vi "json_resolve_key.vi"(11 "key":string) -> (3 "resolved key":string)   [LabVIEW 2017]
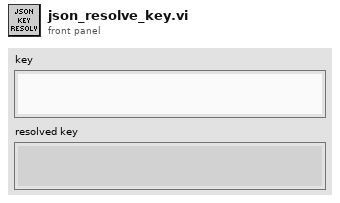
[diagram p1: front panel]
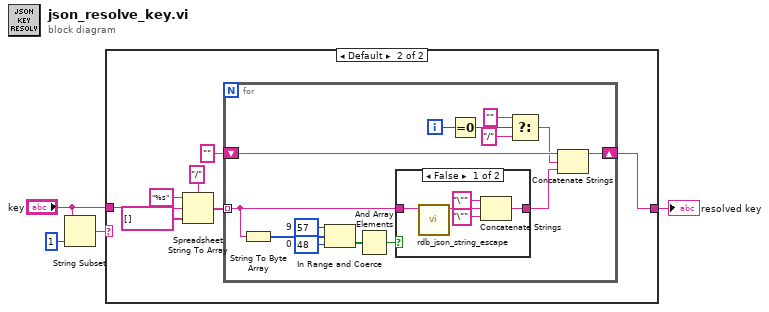
[diagram p0: block diagram]
diagram:
  n1 = String Subset(string="key", length (rest)=1 ("length (rest)")) -> (substring=w3:string)  [unwired: 1 in]
  n2 = case shown="Default" w3 {
    tunnel: "key" -> [w5 w9]
    tunnel: [w5 w6] -> w2
    frame "\"" {
    }
    frame Default {
      n3 = Spreadsheet String To Array(delimiter (Tab)="/", format string="%s", spreadsheet string=w9, array type (2D Dbl)=string[] []) -> (array=w8:string[])
      n4 = for {
        tunnel: w8 -> [w26] mode=indexing
        shift-right: [w18] -> w6
        shift-left: "" -> [w20]
        i -> [w17]
        w25 = u8 48  # 0
        w24 = u8 57  # 9
        n5 = String To Byte Array(string=w26) -> (unsigned byte array=w21:u8[])
        n6 = In Range and Coerce(upper limit=w24, x=w21, lower limit=w25) -> (In Range?=w23:bool[])  [unwired: 1 out]
        n7 = And Array Elements(Boolean array=w23) -> (logical AND=w22:bool)
        n8 = case shown="False" w22 {
          tunnel: w26 -> [w31 w32]
          tunnel: [w27 w32] -> w19
          frame False {
            n9 = call "rdb_json_string_escape.vi"("string"=w31) -> ("escaped string"=w30:string)  [unwired: 10 in]
            n10 = Concatenate Strings("\"" ("string"), w30, "\"" ("string")) -> (w27:string)
          }
          frame True {
            # "number"
          }
        }
        n11 = Equal To 0?(x=w17) -> (x = 0?=w16:bool)
        n12 = Select(t="", s=w16, f="/") -> (s? t:f=w13:string)
        n13 = Concatenate Strings(w20, w13, w19) -> (w18:string)
      }
    }
  }
  "resolved key" <- w2
